vi "Odometry.vi"(8 "L":dbl=100.0 format="%#_13g", 9 "POS in":cluster{"X":dbl, "Y":dbl, "Angle":dbl}, 11 "ENC Diff(mm)":T1) -> (1 "POS out":cluster{"X":dbl, "Y":dbl, "Angle":dbl})   [LabVIEW 2018]
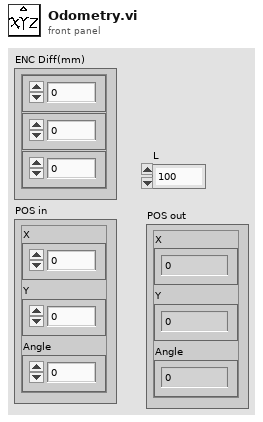
[diagram p1: front panel]
types:
  T1 = cluster{"Numeric Control":dbl, "Numeric Control":dbl, "Numeric Control":dbl}
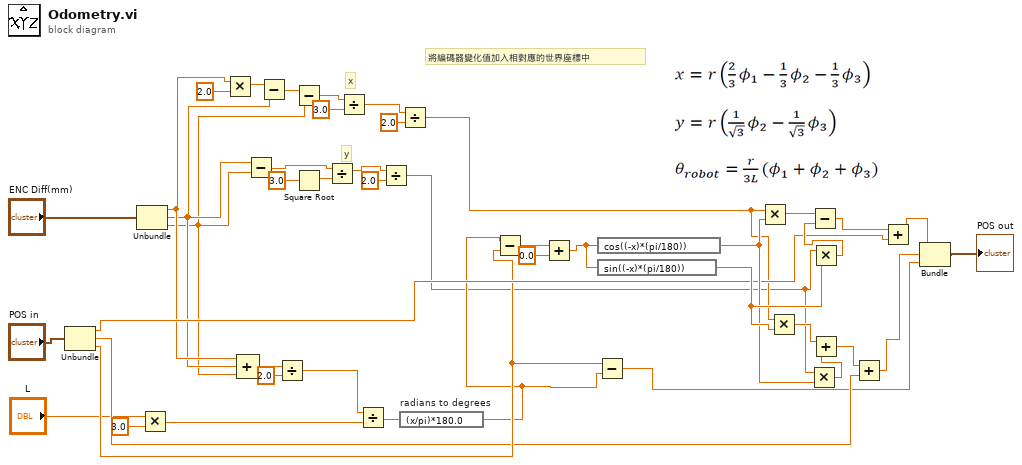
[diagram p0: block diagram]
diagram:
  # "y"
  # "x"
  # "將編碼器變化值加入相對應的世界座標中"
  n1 = Unbundle("POS in") -> ("X"=w34:dbl, "Y"=w31:dbl, "Angle"=w32:dbl)
  n2 = Unbundle("ENC Diff(mm)") -> ("Numeric Control"=w19:dbl, "Numeric Control"=w18:dbl, "Numeric Control"=w17:dbl)
  n3 = Multiply(x="L", y=3.0) -> (x*y=w16:dbl)
  n4 = Multiply(x=w19, y=2.0) -> (x*y=w27:dbl)
  n5 = Compound Arithmetic op=ADD(w19, w18, w17) -> (w9:dbl)
  n6 = Subtract(x=w18, y=w17) -> (x-y=w24:dbl)
  n7 = Subtract(x=w27, y=w18) -> (x-y=w28:dbl)
  n8 = Divide(x=w9, y=2.0) -> (x/y=w7:dbl)
  n9 = Subtract(x=w28, y=w17) -> (x-y=w26:dbl)
  n10 = Square Root(x=3.0) -> (sqrt(x)=w23:dbl)
  n11 = Divide(x=w24, y=w23) -> (x/y=w4:dbl)
  n12 = Divide(x=w26, y=3.0) -> (x/y=w3:dbl)
  n13 = Divide(x=w7, y=w16) -> (x/y=w15:dbl)
  n14 = Divide(x=w4, y=2.0) -> (x/y=w1:dbl)
  n15 = Divide(x=w3, y=2.0) -> (x/y=w2:dbl)
  n16 = expression code="(x/pi)*180.0" "radians to degrees"(w15) -> (w13:dbl)
  n17 = Subtract(x=w13, y=w32) -> (x-y=w12:dbl)
  n18 = Add(x=w12, y=0.0) -> (x+y=w10:dbl)
  n19 = Subtract(x=w32, y=w13) -> (x-y=w14:dbl)
  n20 = expression code="cos((-x)*(pi/180))"(w10) -> (w44:dbl)
  n21 = expression code="sin((-x)*(pi/180))"(w10) -> (w45:dbl)
  n22 = Multiply(x=w2, y=w44) -> (x*y=w43:dbl)
  n23 = Multiply(x=w2, y=w45) -> (x*y=w42:dbl)
  n24 = Multiply(x=w1, y=w44) -> (x*y=w40:dbl)
  n25 = Multiply(x=w1, y=w45) -> (x*y=w41:dbl)
  n26 = Subtract(x=w43, y=w41) -> (x-y=w36:dbl)
  n27 = Add(x=w42, y=w40) -> (x+y=w39:dbl)
  n28 = Add(x=w39, y=w31) -> (x+y=w37:dbl)
  n29 = Add(x=w36, y=w34) -> (x+y=w38:dbl)
  n30 = Bundle(w38, w37, w14) -> (→"POS out":cluster{dbl, dbl, dbl})  [unwired: 1 in]
